vi "Set Control Disabled State (SubVI).vi"(0 "Control Refs":cluster{"Label Name":string, "Ref":refnum<vi>}[](array[cluster]), 5 "Control Names":string[](array[string])=["CONFIG", "START", "STOP", "EMAIL"], 11 "Error IN":errorcluster, 13 "Disable Status":T1(array[ring])) -> (15 "Error OUT":errorcluster)   [LabVIEW 2012]
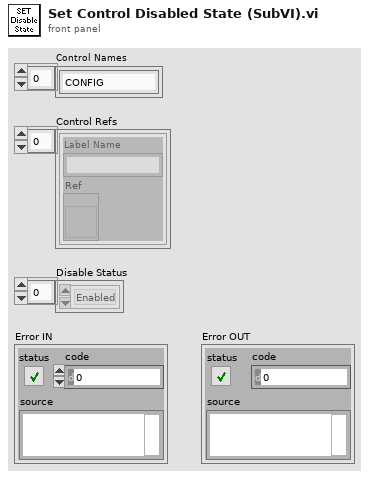
[diagram p1: front panel]
types:
  T1 = enum8{"Enabled", "Disabled", "Disabled and Grayed Out"}[]
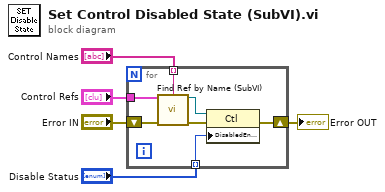
[diagram p0: block diagram]
diagram:
  n1 = for {
    tunnel: "Control Names" -> [w12] mode=indexing
    tunnel: "Control Refs" -> [w11]
    shift-right: [w7] -> w4
    shift-left: "Error IN" -> [w10]
    tunnel: "Disable Status" -> [w6] mode=indexing
    n2 = call "Find Ref by Name (SubVI).vi"("Control Refs"=w11, "Label Name"=w12, "Error IN"=w10) -> ("Control Reference"=w8:refnum<vi>, "Error OUT"=w9:errorcluster)  [unwired: 11 in]
    n3 = property class="Ctl"(reference=w8, error in=w9, "DisabledEnum"=w6) -> (error out=w7:errorcluster)  [unwired: 1 out]
  }
  "Error OUT" <- w4
